vi "GFITS_IMLOG.vi"(6 "max bytes size":i32=200000, 8 "log":bool, 9 "command":string, 10 "imlogpath":path) -> (0 "log out":bool, 2 "answer":string, 3 "imlogpath out":path)   [LabVIEW 2016]
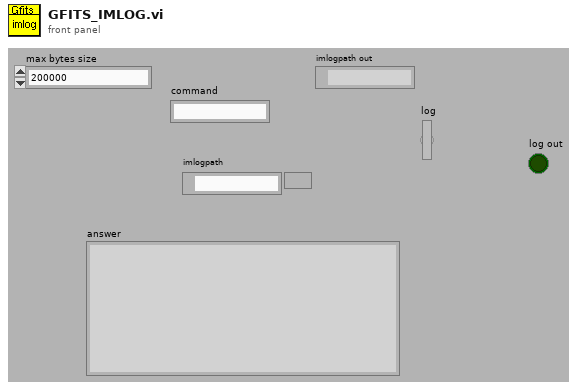
[diagram p1: front panel]
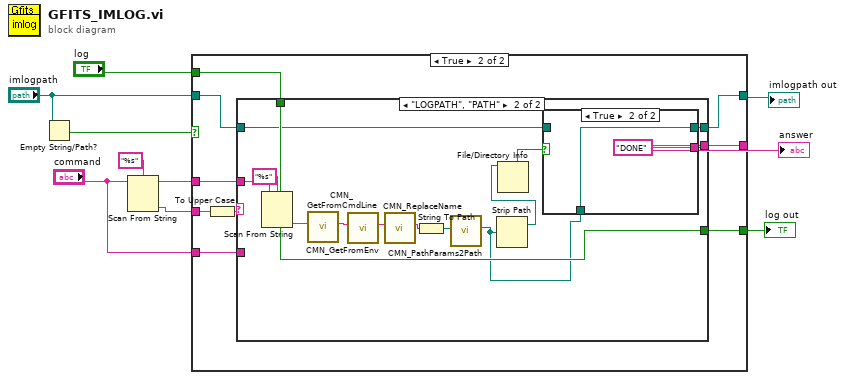
[diagram p0: block diagram]
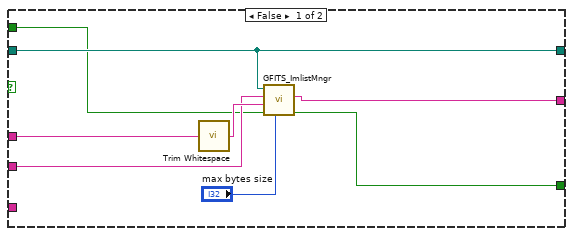
[diagram p2: hidden frame]
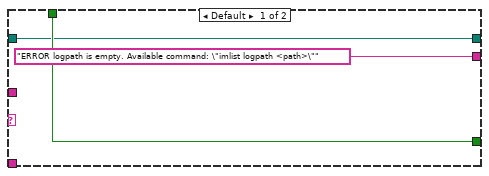
[diagram p3: hidden frame]
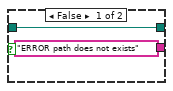
[diagram p4: hidden frame]
diagram:
  n1 = Empty String/Path?(string/path="imlogpath") -> (empty?=w2:bool)
  n2 = Scan From String(format string="%s", input string="command") -> (remaining string=w6:string, output 1=w5:string)  [unwired: 2 in, 3 out]
  n3 = case shown="True" w2 {
    tunnel: "imlogpath" -> [w15 w21]
    tunnel: [w17 w27] -> w9
    tunnel: [w15 w20] -> w8
    tunnel: w6 -> [w14 w19]
    tunnel: w5 -> [w13 w26]
    tunnel: [w11 w24] -> w4
    tunnel: "log" -> [w12 w23]
    tunnel: "command" -> [_ w22]
    frame False {
      n4 = call <vilib>:"Trim Whitespace.vi"("string"=w14) -> ("trimmed string"=w18:string)  [unwired: 1 in]
      n5 = call "GFITS_ImlistMngr.vi"("max bytes size"="max bytes size", "log"=w12, "arguments"=w18, "command"=w13, "images_witten_path"=w15) -> ("log out"=w11:bool, "answer"=w17:string)  [unwired: 5 out]
    }
    frame True {
      n6 = To Upper Case(1:w26) -> (0:w25:string)
      n7 = case shown="\"LOGPATH\", \"PATH\"" w25 {
        tunnel: ["ERROR logpath is empty. Available command: \"imlist logpath <path>\"" w33] -> w27
        tunnel: [w30 w39] -> w24
        tunnel: w23 -> [w30 w39]
        tunnel: w22 -> [_ _]
        tunnel: w21 -> [w29 w32]
        tunnel: [w29 w34] -> w20
        tunnel: w19 -> [_ w43]
        frame Default {
        }
        frame "LOGPATH", "PATH" {
          n8 = Scan From String(format string="%s", input string=w43) -> (output 1=w42:string)  [unwired: 2 in, 4 out]
          n9 = call "CMN_GetFromCmdLine.vi"("str in"=w42) -> ("str out"=w41:string)  [unwired: 10 out]
          n10 = call "CMN_GetFromEnv.vi"("str in"=w41) -> ("str out"=w40:string)  [unwired: 10 out]
          n11 = call "CMN_ReplaceName.vi"("name in"=w40) -> ("name out"=w38:string)  [unwired: 1 in, 9 out]
          n12 = String To Path(string=w38) -> (path=w37:path)
          n13 = call "CMN_PathParams2Path.vi"("Path In"=w37) -> ("Path out"=w31:path)  [unwired: 2 in, 8 out]
          n14 = Strip Path(path=w31) -> (stripped path=w35:path)  [unwired: 1 out]
          n15 = File/Directory Info(path=w35) -> (directory=w36:bool)  [unwired: 1 in, 6 out]
          n16 = case shown="True" w36 {
            tunnel: w31 -> [_ w48]
            tunnel: [w46 w48] -> w34
            tunnel: ["ERROR path does not exists" "DONE"] -> w33
            tunnel: w32 -> [w46 _]
            frame False {
            }
            frame True {
            }
          }
        }
      }
    }
  }
  "answer" <- w9
  "imlogpath out" <- w8
  "log out" <- w4
